vi "Deep-Diver.vi"() -> ()   [LabVIEW 2020]
panel:
  out "Image":picture
  out "File (Image)":string
  in  "Next Image":bool
  in  "Prev Image":bool
  out "Occurrence":string
  out "Type":string
  out "DOCX":i32
  out "ZIP":i32
  in  "Next Context":bool
  in  "Prev Context":bool
  out "Context":string
  out "File (Text)":string
  out "Occurrences":dbl
  out "Selected Word":string[](array[string])
  out "JPG":i32
  out "PNG":i32
  in  "Context Length (Chars)":dbl
  in  "Words to Search":path
  in  "Start Button":bool
  in  "DOCX":bool=TRUE
  in  "ZIP":bool=TRUE
  in  "JPG":bool=TRUE
  in  "PNG":bool=TRUE
  in  "File/Directory":path
  in  "Stop":bool
  # "File/Directory"
  # "Text Found"
  # "Image Preview"
  # "Configuration"
  # "Searching for File Types:"
  # "Text Search Options:"
  # "Words to Search (TXT)"
  # "File Information"
  # "Number of Files Found:"
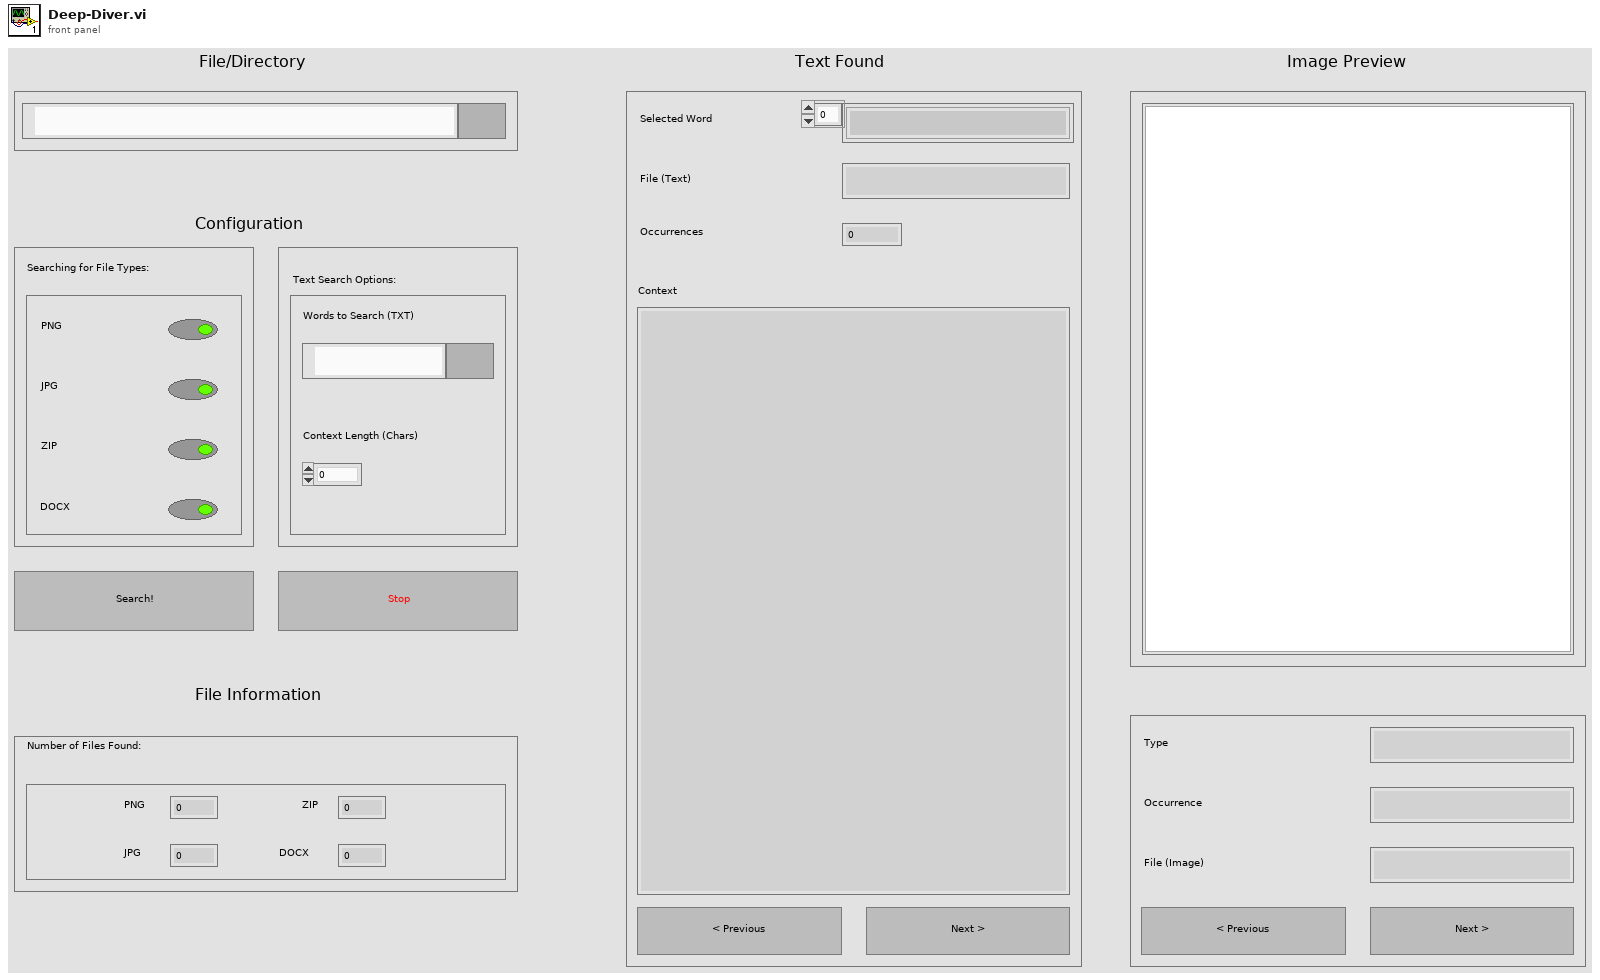
[diagram p1: front panel]
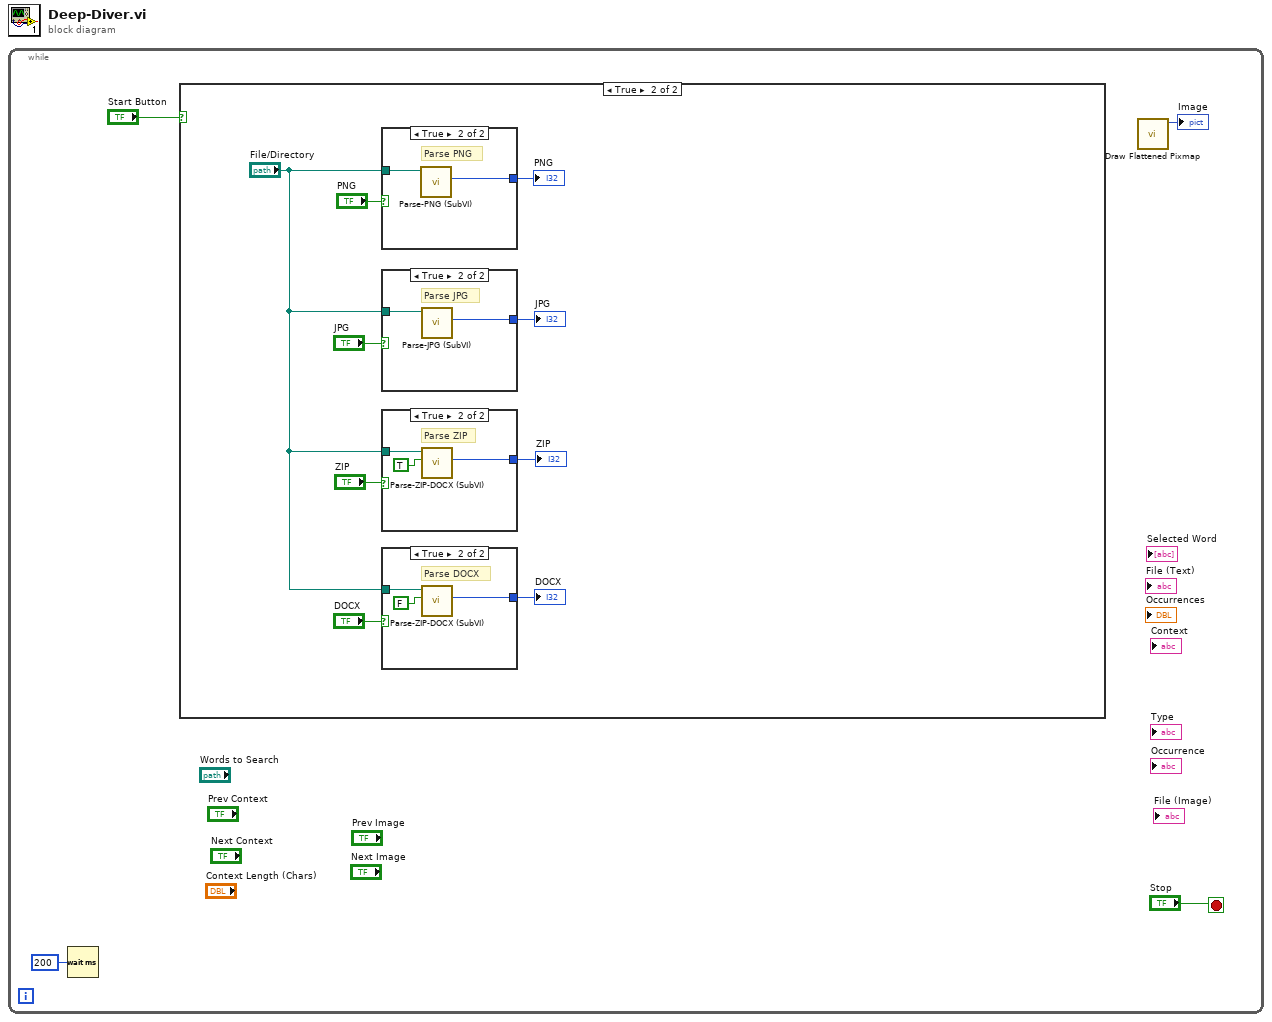
[diagram p0: block diagram]
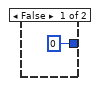
[diagram p3: hidden frame]
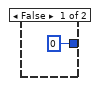
[diagram p4: hidden frame]
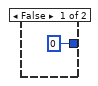
[diagram p5: hidden frame]
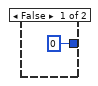
[diagram p6: hidden frame]
diagram:
  n1 = while {
    stop <- "Stop" stop-if-true
    n2 = Wait (ms)(milliseconds to wait=u32 200) -> ()  [unwired: 1 out]
    n3 = case shown="True" "Start Button" {
      frame False {
      }
      frame True {
        n4 = case shown="True" "PNG" {
          tunnel: "File/Directory" -> [_ w27]
          tunnel: [0 ("Files Found") w26] -> w8
          frame False {
          }
          frame True {
            # "Parse PNG"
            n5 = call "Parse-PNG (SubVI).vi"("Unknown File"=w27) -> ("Files Found"=w26:i32)  [unwired: 9 in, 1 out]
          }
        }
        "PNG" <- w8
        n6 = case shown="True" "JPG" {
          tunnel: "File/Directory" -> [_ w24]
          tunnel: [0 ("Files Found") w23] -> w7
          frame False {
          }
          frame True {
            # "Parse JPG"
            n7 = call "Parse-JPG (SubVI).vi"("Unknown File"=w24) -> ("Files Found"=w23:i32)  [unwired: 9 in, 1 out]
          }
        }
        "JPG" <- w7
        n8 = case shown="True" "ZIP" {
          tunnel: "File/Directory" -> [_ w21]
          tunnel: [0 ("Files Found") w19] -> w6
          frame False {
          }
          frame True {
            # "Parse ZIP"
            n9 = call "Parse-ZIP-DOCX (SubVI).vi"("Is ZIP"=TRUE, "Unknown File"=w21) -> ("Files Found"=w19:i32)  [unwired: 8 in, 1 out]
          }
        }
        "ZIP" <- w6
        n10 = case shown="True" "DOCX" {
          tunnel: "File/Directory" -> [_ w17]
          tunnel: [0 ("Files Found") w15] -> w5
          frame False {
          }
          frame True {
            # "Parse DOCX"
            n11 = call "Parse-ZIP-DOCX (SubVI).vi"("Is ZIP"=FALSE, "Unknown File"=w17) -> ("Files Found"=w15:i32)  [unwired: 8 in, 1 out]
          }
        }
        "DOCX" <- w5
      }
    }
    n12 = call <vilib>:"Draw Flattened Pixmap.vi"() -> ("new picture"=→"Image":picture)  [unwired: 9 in]
  }
